vi "Save Ramp Time.vi"(0 "section":string, 1 "Input Cluster":T1, 2 "refnum":T2, 3 "error in (no error)":errorcluster, 4 "Ramp Type String":string) -> (6 "refnum out":T2, 7 "error out":errorcluster)   [LabVIEW 2009]
uses:
  <vilib>/Utility/config.llb/Config Data RefNum.ctl
  MixedMode/Ramp Control.ctl
  <vilib>/Utility/config.llb/Write Key (Double).vi
  <vilib>/Utility/config.llb/NI_LVConfig.lvlib
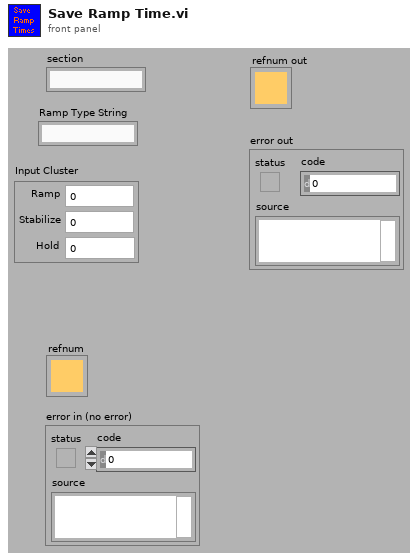
[diagram p1: front panel]
types:
  T1 = typedef "Ramp Control.ctl" = cluster{"Ramp":dbl, "Stabilize":dbl, "Hold":dbl}
  T2 = typedef "NI_LVConfig.lvlib/Config Data RefNum.ctl" = refnum<k1>
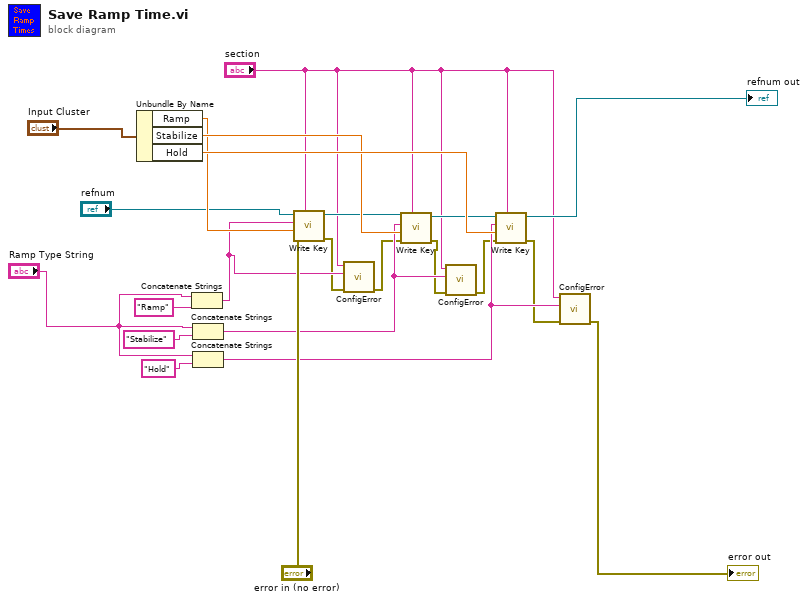
[diagram p0: block diagram]
diagram:
  n1 = Unbundle By Name("Input Cluster") -> ("Ramp"=w18:dbl, "Stabilize"=w21:dbl, "Hold"=w23:dbl)
  n2 = Concatenate Strings("Ramp Type String", "Ramp" ("string")) -> (w4:string)
  n3 = Concatenate Strings("Ramp Type String", "Stabilize" ("string")) -> (w8:string)
  n4 = Concatenate Strings("Ramp Type String", "Hold" ("string")) -> (w11:string)
  n5 = call-poly <vilib>:"Write Key.vi"("section"="section", "error in (no error)"="error in (no error)", "value"=w18, "key"=w4, "refnum"="refnum") -> ("error out"=w3:errorcluster, "refnum out"=w20:T2)  [unwired: 3 in, 2 out]
  n6 = call "ConfigError.vi"("error in (no error)"=w3, "Key"=w4, "Section"="section") -> ("error out"=w2:errorcluster)  [unwired: 8 out]
  n7 = call-poly <vilib>:"Write Key.vi"("section"="section", "error in (no error)"=w2, "value"=w21, "key"=w8, "refnum"=w20) -> ("error out"=w7:errorcluster, "refnum out"=w22:T2)  [unwired: 3 in, 2 out]
  n8 = call "ConfigError.vi"("error in (no error)"=w7, "Key"=w8, "Section"="section") -> ("error out"=w6:errorcluster)  [unwired: 8 out]
  n9 = call-poly <vilib>:"Write Key.vi"("section"="section", "error in (no error)"=w6, "value"=w23, "key"=w11, "refnum"=w22) -> ("error out"=w10:errorcluster, "refnum out"=→"refnum out":T2)  [unwired: 3 in, 2 out]
  n10 = call "ConfigError.vi"("error in (no error)"=w10, "Key"=w11, "Section"="section") -> ("error out"=→"error out":errorcluster)  [unwired: 8 out]
